vi "LaudaLedCtrl.vi"(9 "Manual select":T1(radio), 10 "T ext / T ext in":enum32{"Sensor 1", "Sensor 2"}(radio), 11 "Lauda port":dbl) -> (1 "Sensor OK 5":bool, 2 "Sensor OK 3":bool, 3 "Sensor OK 4":bool, 4 "Sensor OK 6":bool)   [LabVIEW 2016]
uses:
  x64/Debug/BERTTA.dll
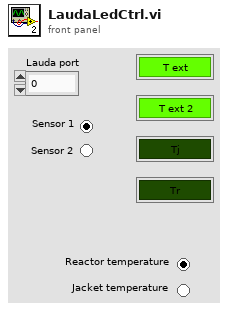
[diagram p1: front panel]
types:
  T1 = enum32{"Reactor temperature", "Jacket temperature"}
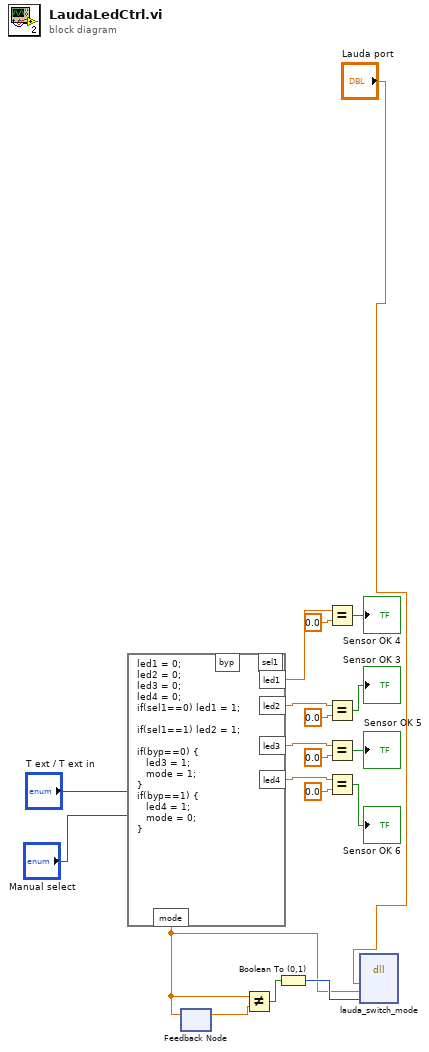
[diagram p0: block diagram]
diagram:
  n1 = formula code="led1 = 0;\nled2 = 0;\nled3 = 0;\nled4 = 0;\nif(sel1==0) led1 = 1;\n\nif(sel1==1) led2 = 1;\n\nif(byp==0) {\n   led3 = 1;\n   mode = 1;\n}\nif(byp==1) {\n   led4 = 1;\n   mode = 0;\n}"("sel1"="T ext / T ext in", "byp"="Manual select") -> ("led1"=w2:dbl, "led2"=w4:dbl, "led3"=w9:dbl, "led4"=w10:dbl, "mode"=w15:dbl)
  n2 = feedback #1() -> (w16:dbl)  [unwired: 1 in]
  n3 = feedback-in #1(w15) -> ()
  n4 = Not Equal?(x=w15, y=w16) -> (x != y?=w18:bool)
  n5 = Boolean To (0,1)(Boolean=w18) -> (0, 1=w17:i16)
  n6 = Equal?(x=w2, y=0.0) -> (x = y?=→"Sensor OK 4":bool)
  n7 = Equal?(x=w4, y=0.0) -> (x = y?=→"Sensor OK 3":bool)
  n8 = Equal?(x=w9, y=0.0) -> (x = y?=→"Sensor OK 5":bool)
  n9 = Equal?(x=w10, y=0.0) -> (x = y?=→"Sensor OK 6":bool)
  n10 = dll-call lib="C:/Users/shresplab/OneDrive - Kemira Oyj/Documents/GitHub/Bertta/BERTTA/x64/Debug/BERTTA.dll" fn="lauda_switch_mode"("port"="Lauda port", "mode"=w15, "enable"=w17) -> ()  [unwired: 7 in, 2 out]
